vi "getSerializedData.vi"(0 "reference":refnum<class "StateNode.lvclass">, 5 "error in (no error)":errorcluster) -> (14 "reference out":refnum<class "StateNode.lvclass">, 15 "parent":refnum<class "AbstractNode.lvclass">, 16 "children":refnum<class "AbstractNode.lvclass">[](array[class]), 17 "xmlOut":string, 19 "error out":errorcluster)   [LabVIEW 2016, in "StateNode.lvclass"]
doc: "getSerializedData"
uses:
  <resource>/Framework/Providers/Open_GDS/UML/StateNode_class/StateNode.lvclass
  C:/Program Files (x86)/National Instruments/LabVIEW 2016/resource/Framework/Providers/Open_GDS/UML/RectangularNode_class/RectangularNode.lvclass
  C:/Program Files (x86)/National Instruments/LabVIEW 2016/resource/Framework/Providers/Open_GDS/UML/AbstractNode_class/AbstractNode.lvclass
  <resource>/Framework/Providers/Open_GDS/UML/AbstractNode_class/AbstractNode.lvclass
  <resource>/Framework/Providers/Open_GDS/UML/General/Rectangle/Rectangle Rectangle2D.ctl
  <resource>/Framework/Providers/Open_GDS/UML/MultiLineString_class/MultiLineString.lvclass
  <resource>/Framework/Providers/Open_GDS/UML/RectangularNode_class/RectangularNode.lvclass
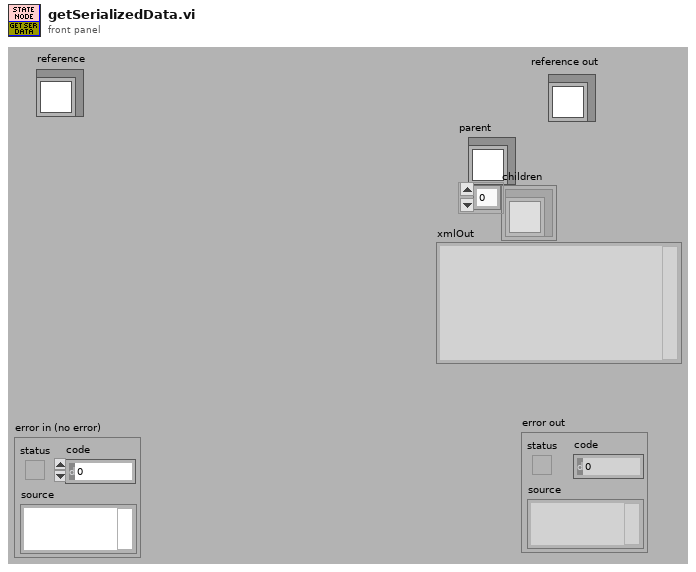
[diagram p1: front panel]
types:
  T1 = typedef "Rectangle Rectangle2D.ctl" = cluster{"x":dbl, "y":dbl, "width":dbl, "height":dbl}
  T2 = cluster{"Base class":cluster{"Base class":cluster{"parent":refnum<k1>, "children":refnum<k1>[]}, "bounds":T1}, "state":refnum<k1>, "action":refnum<k1>, "DEFAULT_WIDTH":i32, "DEFAULT_HEIGHT":i32}
  T3 = typedef "StateNode.lvclass/ObjectAttributes.ctl" = cluster{"state":refnum<class "MultiLineString.lvclass">, "action":refnum<class "MultiLineString.lvclass">, "DEFAULT_WIDTH":i32, "DEFAULT_HEIGHT":i32}
  T4 = typedef "RectangularNode.lvclass/ObjectAttributes.ctl" = cluster{"bounds":T1}
  T5 = typedef "AbstractNode.lvclass/ObjectAttributes.ctl" = cluster{"parent":refnum<class "AbstractNode.lvclass">, "children":refnum<class "AbstractNode.lvclass">[], "Hidden":bool}
  T6 = cluster{"Attributes":cluster{"Base class":cluster{"Base class":cluster{"parent":refnum<k1>, "children":refnum<k1>[]}, "bounds":T1}, "state":refnum<k1>, "action":refnum<k1>, "DEFAULT_WIDTH":i32, "DEFAULT_HEIGHT":i32}, "text":string, "text":string}
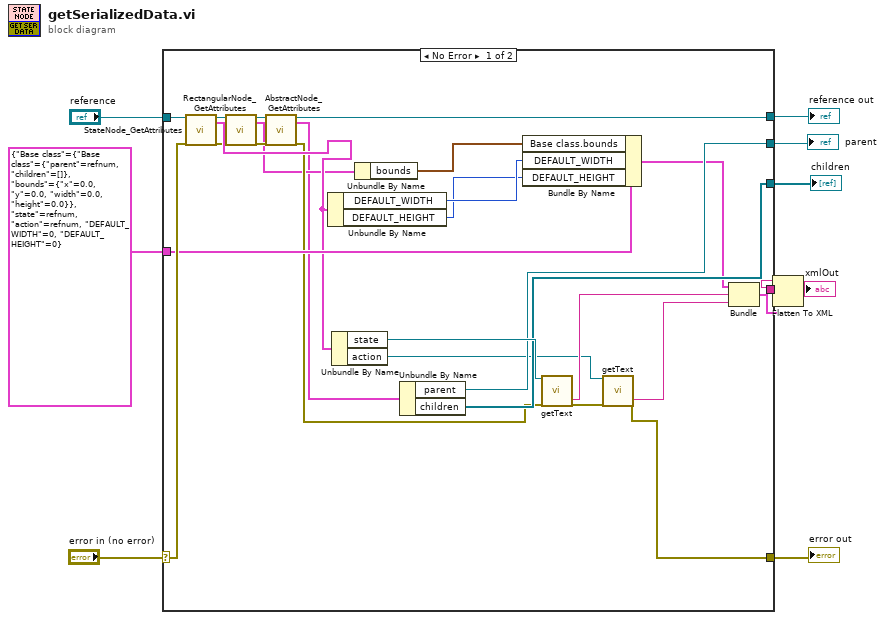
[diagram p0: block diagram]
diagram:
  n1 = case shown="No Error" "error in (no error)" {
    selector: "error in (no error)" -> [w34 w35]
    tunnel: "reference" -> [w33 w36]
    tunnel: [w25 w35] -> w6
    tunnel: [w11 w36] -> w5
    tunnel: [w29 _] -> w4
    tunnel: [w28 _] -> w3
    tunnel: [w27 _] -> w2
    tunnel: T2 {"Base class"={"Base class"={"parent"=refnum, "children"=[]}, "bounds"={"x"=0.0, "y"=0.0, "width"=0.0, "height"=0.0}}, "state"=refnum, "action"=refnum, "DEFAULT_WIDTH"=0, "DEFAULT_HEIGHT"=0} ("Attributes") -> [w19 _]
    frame No Error {
      n2 = call <resource>:"StateNode_GetAttributes.vi"("reference in"=w33, "error in (no error)"=w34) -> ("reference out"=w16:refnum<class "StateNode.lvclass">, "Data"=w17:T3, "error out"=w15:errorcluster)  [unwired: 1 in, 14 out]
      n3 = call <resource>:"RectangularNode_GetAttributes.vi"("reference in"=w16, "error in (no error)"=w15) -> ("reference out"=w14:refnum<class "StateNode.lvclass">, "Data"=w10:T4, "error out"=w13:errorcluster)  [unwired: 14 in, 1 out]
      n4 = call <resource>:"AbstractNode_GetAttributes.vi"("reference in"=w14, "error in (no error)"=w13) -> ("reference out"=w11:refnum<class "StateNode.lvclass">, "Data"=w9:T5, "error out"=w12:errorcluster)  [unwired: 14 in, 1 out]
      n5 = Unbundle By Name(w17) -> ("DEFAULT_WIDTH"=w21:i32, "DEFAULT_HEIGHT"=w20:i32)
      n6 = Unbundle By Name(w17) -> ("state"=w31:refnum<class "MultiLineString.lvclass">, "action"=w24:refnum<class "MultiLineString.lvclass">)
      n7 = Unbundle By Name(w10) -> ("bounds"=w22:T1)
      n8 = Unbundle By Name(w9) -> ("parent"=w29:refnum<class "AbstractNode.lvclass">, "children"=w28:refnum<class "AbstractNode.lvclass">[])
      n9 = Bundle By Name(cluster=w19, "Base class.bounds"=w22, "DEFAULT_WIDTH"=w21, "DEFAULT_HEIGHT"=w20) -> (w18:T2)
      n10 = call-dynamic "getText.vi"("reference"=w31, "error in (no error)"=w12) -> ("text"=w30:string, "error out"=w26:errorcluster)  [unwired: 16 out]
      n11 = call-dynamic "getText.vi"("reference"=w24, "error in (no error)"=w26) -> ("text"=w23:string, "error out"=w25:errorcluster)  [unwired: 16 out]
      n12 = Bundle("Attributes"=w18, "text"=w30, "text"=w23) -> (w32:T6)  [unwired: 1 out]
      n13 = Flatten To XML(anything=w32) -> (xml string=w27:string)
    }
    frame Error {
    }
  }
  "reference out" <- w5
  "error out" <- w6
  "parent" <- w4
  "children" <- w3
  "xmlOut" <- w2
